vi "Data_Filtering_and_Processing Log.vi"() -> ()   [LabVIEW 2020]
uses:
  Global Variables/Training_Status.vi
  Global Variables/Number_of_Windows.vi
  Global Variables/Trial_Flag.vi
  Global Variables/Global Enable Logging.vi
panel:
  out "Array out":sgl[](array[numeric])
  out "Sended frame":dbl[](array[numeric])
  in  "stop":bool
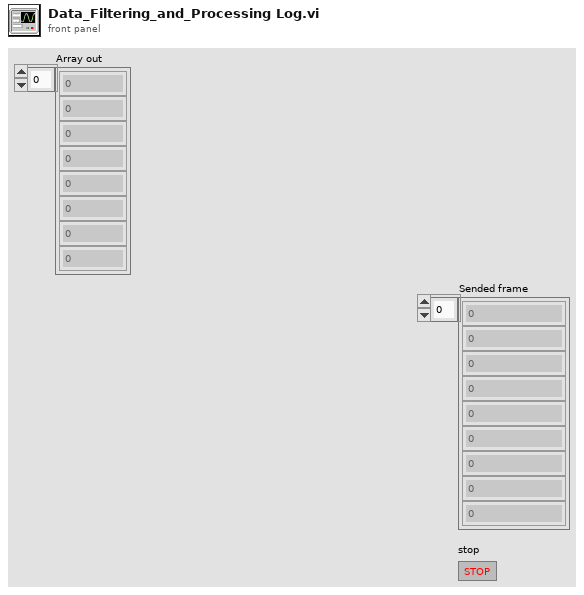
[diagram p1: front panel]
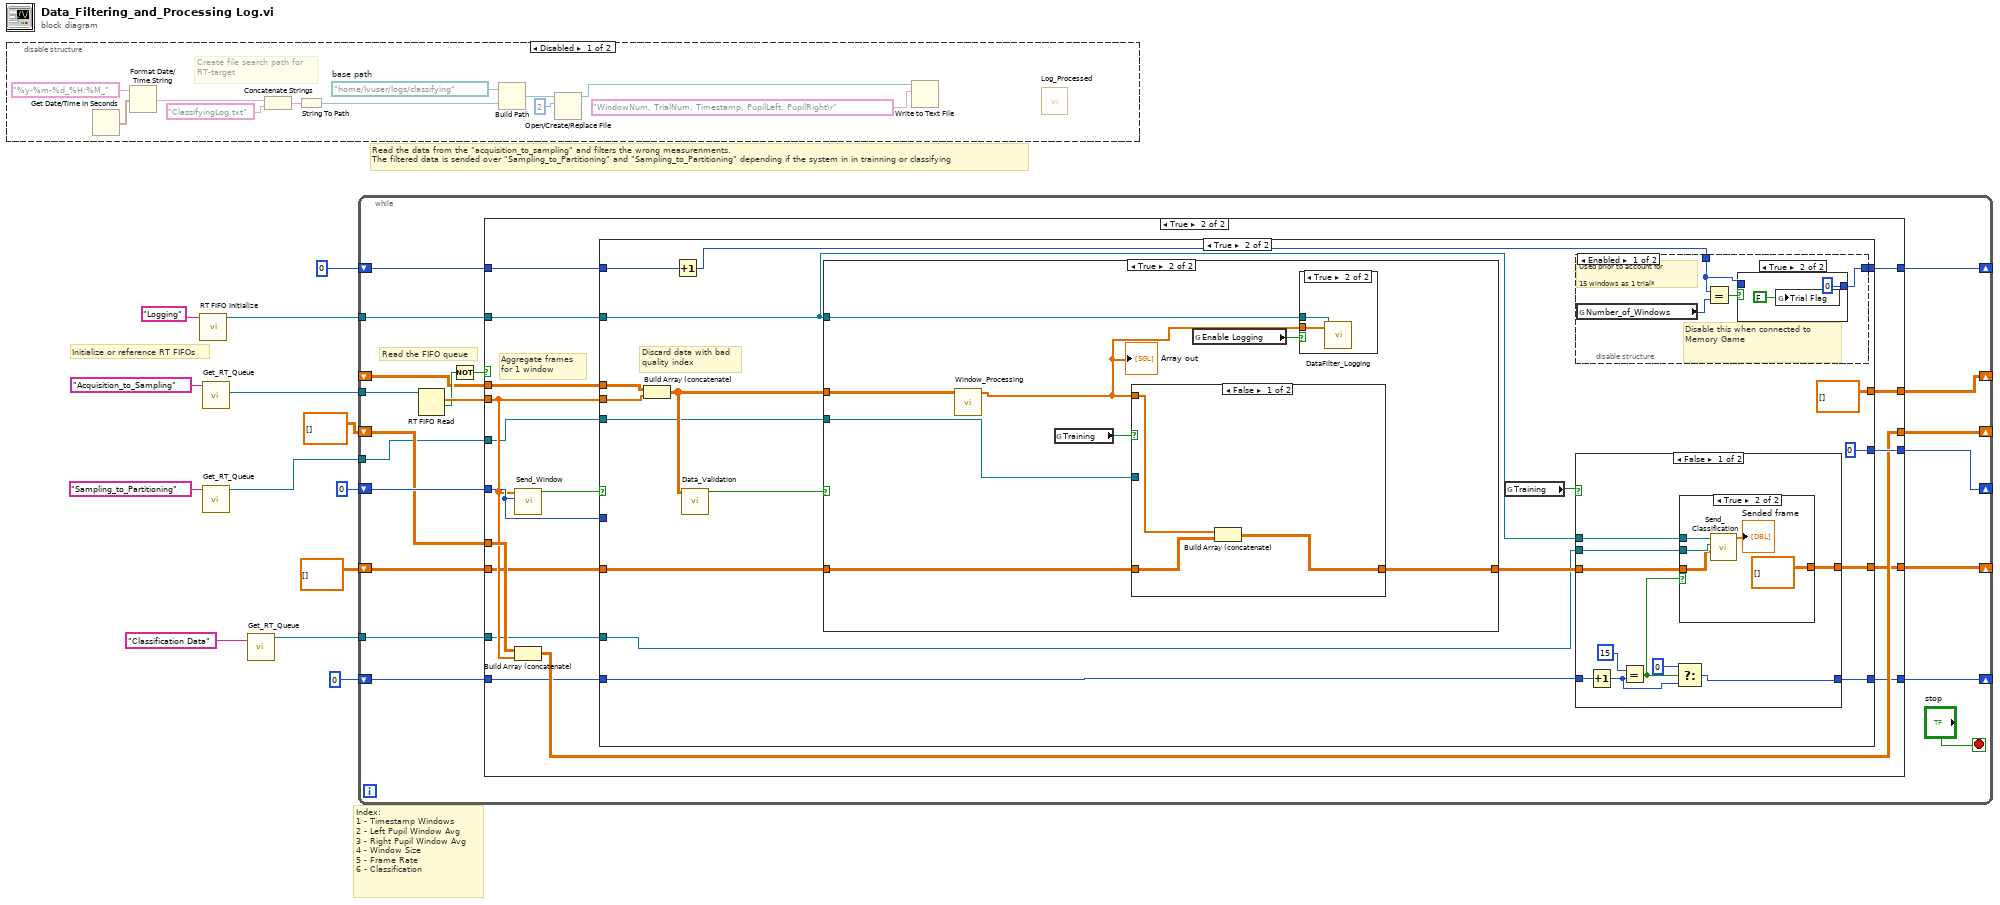
[diagram p0: block diagram]
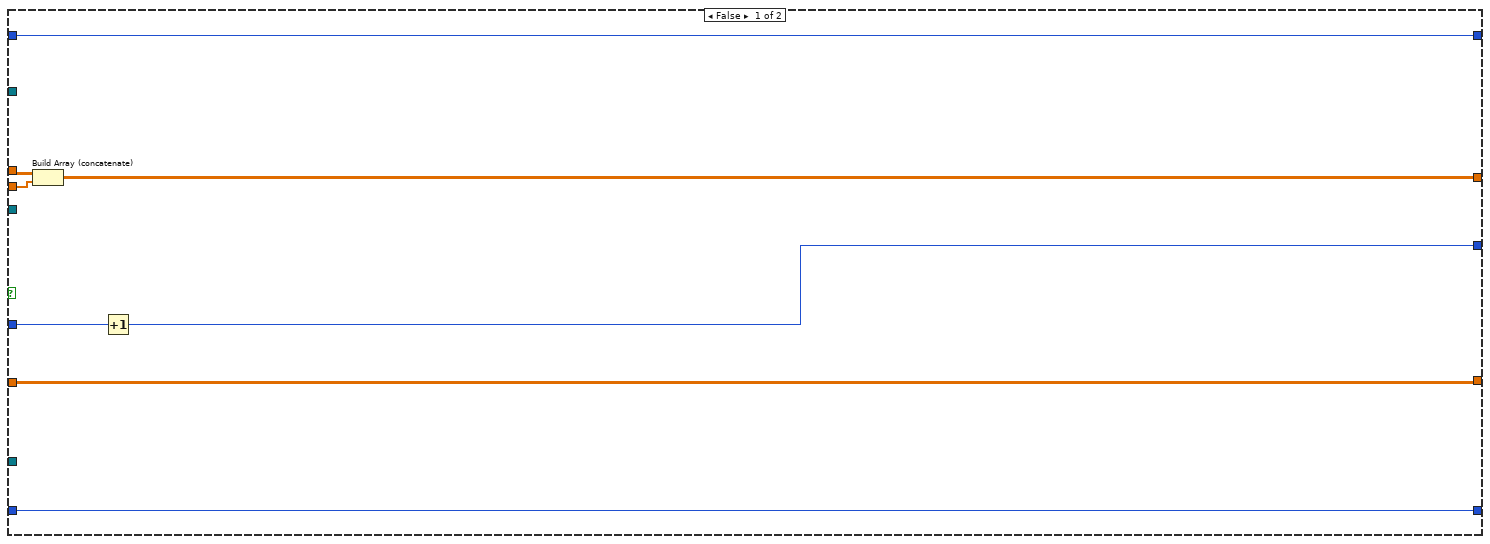
[diagram p4: hidden frame]
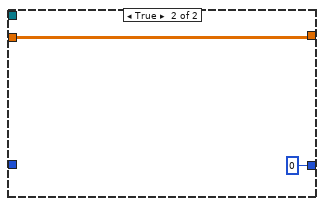
[diagram p6: hidden frame]
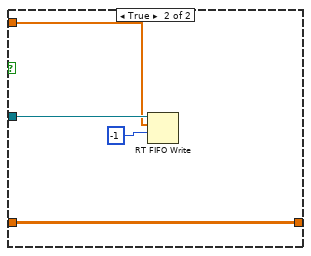
[diagram p11: hidden frame]
diagram:
  # "Index: \n1 - Timestamp Windows \n2 - Left Pupil Window Avg \n3 - Right Pupil Window Avg\n4 - Window Size\n5 - Frame Rate\n6 - Classification"
  # "Initialize or reference RT FIFOs"
  # "Read the data from the \"acquisition_to_sampling\" and filters the wrong measurenments. \nThe filtered data is sended over \"Sampling_to_Partitioning\" and \"Sampling_to_Partitioning\" depending if the system in in trainning or classifying"
  n1 = disable-structure shown="Disabled" {
    frame Disabled {
      w23 = path "/home/lvuser/logs/classifying"  # base path
      # "Create file search path for \nRT-target"
      n2 = Get Date/Time In Seconds() -> (seconds since 1Jan1904=w18:timestamp)
      n3 = Format Date/Time String(time format string (%c)="%y-%m-%d_%H:%M_", seconds (now)=w18) -> (date/time string=w17:string)  [unwired: 1 in]
      n4 = Concatenate Strings(w17, "ClassifyingLog.txt") -> (w20:string)
      n5 = String To Path(string=w20) -> (path=w21:path)
      n6 = Build Path(base path=w23, name or relative path=w21) -> (appended path=w24:path)
      n7 = Open/Create/Replace File(file path (use dialog)=w24, operation (0:open)=2) -> (refnum out=w14:refnum<file>)  [unwired: 4 in, 2 out]
      n8 = Write to Text File(file (use dialog)=w14, text="WindowNum, TrialNum, Timestamp, PupilLeft, PupilRight\r") -> ()  [unwired: 2 in, 3 out]
      n9 = call "Log_Processed.vi"() -> ()  [unwired: 11 in, 1 out]
    }
    frame Enabled {
    }
  }
  n10 = call "RT FIFO Initialize.vi"("name (unnamed)"="Logging") -> ("rt fifo"=w6:refnum<k33>)  [unwired: 9 in, 1 out]
  n11 = call "Get_RT_Queue.vi"("String"="Acquisition_to_Sampling") -> ("rt fifo double"=w8:refnum<k33>)  [unwired: 8 in, 2 out]
  n12 = call "Get_RT_Queue.vi"("String"="Sampling_to_Partitioning") -> ("rt fifo single"=w11:refnum<k33>)  [unwired: 8 in, 2 out]
  n13 = call "Get_RT_Queue.vi"("String"="Classification Data") -> ("rt fifo single"=w2:refnum<k33>)  [unwired: 8 in, 2 out]
  n14 = while {
    shift-right: [w44] -> _
    shift-left: 0 -> [w42]
    shift-right: [w40] -> _
    shift-left: dbl[][] [] -> [w41]
    tunnel: w8 -> [w38]
    tunnel: w11 -> [w35]
    tunnel: w6 -> [w34]
    shift-right: [w31] -> _
    shift-left: 0 -> [w32]
    shift-right: [w30] -> _
    shift-left: sgl[][] [] -> [w33]
    tunnel: w2 -> [w29]
    shift-right: [w27] -> _
    shift-left: _ -> [w28]
    shift-right: [w25] -> _
    shift-left: 0 -> [w26]
    stop <- "stop" stop-if-true
    # "Read the FIFO queue"
    n15 = RT FIFO Read(0:w38) -> (9:w39:dbl[], 10:w37:bool)  [unwired: 3 in, 3 out]
    n16 = Not(x=w37) -> (.not. x?=w36:bool)
    n17 = case shown="True" w36 {
      tunnel: [w50 w67] -> w44
      tunnel: w42 -> [w50 w66]
      tunnel: w39 -> [_ w62]
      tunnel: w41 -> [w49 w64]
      tunnel: [w49 w63] -> w40
      tunnel: w35 -> [_ w61]
      tunnel: w34 -> [_ w60]
      tunnel: w33 -> [w48 w59]
      tunnel: w32 -> [w46 w58]
      tunnel: [w46 w57] -> w31
      tunnel: [w48 w56] -> w30
      tunnel: w29 -> [_ w55]
      tunnel: w28 -> [w47 w54]
      tunnel: [w47 w53] -> w27
      tunnel: w26 -> [w45 w52]
      tunnel: [w45 w51] -> w25
      frame False {
      }
      frame True {
        # "Aggregate frames \nfor 1 window"
        n18 = call "Send_Window.vi"("Iteration"=w66, "Data Sample"=w62) -> ("Boolean"=w65:bool)  [unwired: 9 in]
        n19 = Build Array (concatenate)(w64, w62) -> (w63:dbl[][])
        n20 = case shown="True" w65 {
          tunnel: w66 -> [w75 _]
          tunnel: [w74 0] -> w67
          tunnel: w62 -> [w70 w92]
          tunnel: w61 -> [_ w89]
          tunnel: w60 -> [_ w82]
          tunnel: w59 -> [w73 w88]
          tunnel: w58 -> [w72 w87]
          tunnel: [w72 w85] -> w57
          tunnel: [w73 w83] -> w56
          tunnel: w55 -> [_ w81]
          tunnel: w54 -> [w71 w80]
          tunnel: [w69 dbl[][] []] -> w53
          tunnel: w52 -> [w68 w78]
          tunnel: [w68 w76] -> w51
          frame False {
            n21 = Build Array (concatenate)(w71, w70) -> (w69:dbl[][])
            n22 = Increment(x=w75) -> (x+1=w74:i32)
          }
          frame True {
            # "Discard data with bad\nquality index"
            n23 = Build Array (concatenate)(w80, w92) -> (w91:dbl[][])
            n24 = Increment(x=w78) -> (x+1=w77:i32)
            n25 = call "Data_Validation.vi"("Array"=w91) -> ("Correct Record"=w90:bool)  [unwired: 10 in]
            n26 = case shown="True" w90 {
              tunnel: w91 -> [_ w127]
              tunnel: w89 -> [_ w125]
              tunnel: w82 -> [_ w124]
              tunnel: w88 -> [w119 w122]
              tunnel: [w119 w121] -> w84
              frame False {
              }
              frame True {
                n27 = call "Window_Processing.vi"("Array in"=w127) -> ("Array out"=w120:sgl[])  [unwired: 10 in]
                "Array out" <- w120
                n28 = global read "Training_Status.vi" "Training"() -> (w126:bool)
                n29 = case shown="False" w126 {
                  tunnel: w125 -> [_ w136]
                  tunnel: w120 -> [w131 w134]
                  tunnel: w122 -> [w132 w133]
                  tunnel: [w130 w133] -> w121
                  frame False {
                    n30 = Build Array (concatenate)(w131, w132) -> (w130:sgl[][])
                  }
                  frame True {
                    n31 = RT FIFO Write(0:w136, 1:w134, 2:-1 ("timeout in ms (0)")) -> ()  [unwired: 2 in, 4 out]
                  }
                }
                n32 = global read "Global Enable Logging.vi" "Enable Logging"() -> (w123:bool)
                n33 = case shown="True" w123 {
                  tunnel: w124 -> [_ w129]
                  tunnel: w120 -> [_ w128]
                  frame False {
                  }
                  frame True {
                    n34 = call "DataFilter_Logging.vi"("Input Array"=w128, "rt fifo"=w129) -> ()  [unwired: 9 in, 1 out]
                  }
                }
              }
            }
            n35 = global read "Training_Status.vi" "Training"() -> (w86:bool)
            n36 = disable-structure shown="Enabled" {
              disable-tunnel: w77 -> [w113 _]
              disable-tunnel: [w112 _] -> w76
              frame Enabled {
                # "Used prior to account for \n\n15 windows as 1 trial*"
                # "Disable this when connected to Memory Game"
                n37 = global read "Number_of_Windows.vi" "Number_of_Windows"() -> (w114:i64)
                n38 = Equal?(x=w113, y=w114) -> (x = y?=w115:bool)
                n39 = case shown="True" w115 {
                  tunnel: w113 -> [w116 _]
                  tunnel: [w116 0] -> w112
                  frame False {
                  }
                  frame True {
                    n40 = global write "Trial_Flag.vi" "Trial Flag"(FALSE) -> ()
                  }
                }
              }
              frame Disabled {
              }
            }
            n41 = case shown="False" w86 {
              tunnel: w87 -> [w103 _]
              tunnel: [w99 0 ("t")] -> w85
              tunnel: w84 -> [w97 w111]
              tunnel: [w96 w111] -> w83
              tunnel: w82 -> [w95 _]
              tunnel: w81 -> [w94 _]
              frame False {
                n42 = Increment(x=w103) -> (x+1=w101:i32)
                n43 = Equal?(x=15, y=w101) -> (x = y?=w98:bool)
                n44 = Select(t=0, s=w98, f=w101) -> (s? t:f=w99:i32)
                n45 = case shown="True" w98 {
                  tunnel: w97 -> [w104 w106]
                  tunnel: [w104 sgl[][] []] -> w96
                  tunnel: w95 -> [_ w108]
                  tunnel: w94 -> [_ w107]
                  frame False {
                  }
                  frame True {
                    n46 = call "Send_Classification.vi"("logging FIFO"=w108, "Classification FIFO"=w107, "Window"=w106) -> ("Sended frame"=→"Sended frame":dbl[])  [unwired: 6 in]
                  }
                }
              }
              frame True {
              }
            }
          }
        }
      }
    }
  }
